vi "TB-Config.vi"(0 "Params":T27={"Low cutoff (kHz)"=0.0, "High cutoff (kHz)"=0.0, "Duration (min)"=0.0, "dB SPL"=0.0, "Waveform"=enum."OFF", "WAVfile"=path "", "refWav"=path "", "use mic correction"=FALSE, "micCorrFile"=path "", "Pistonphone Level (dB SPL)"=0.0, "Sampling rate (Hz)"=0.0, "Buffer length (s)"=0.0, "Stream mic"=FALSE, "Fine adjust"={"Max"=0.0, "Min"=0.0}, "Mic gain"=0.0, "atten"=0.0, "resol (Hz)"=0.0, "navgs"=0, "Allow Slack"=FALSE, "max starts"=0, "Freq (kHz)"=8.0, "Tma (s)"=0.0, "Streamed"=[], "Drive"=""}, 1 "Exposure?":bool, 9 "ID":string, 11 "error in (no error)":errorcluster) -> (4 "state":T25, 10 "Num Buffers":i32, 13 "stimulus state":T1, 14 "StimChan":T24 {"Filter"."IIR Filter Cluster"."Forward Coefficients" format="%.4f"; "Filter"."IIR Filter Cluster"."Reverse Coefficients" format="%.4f"}, 15 "error out":errorcluster)   [LabVIEW 2020]
uses:
  Typedefs/TB-Parameters.ctl
  epl-vi-lib/Signal Synthesis VIs/Controls/Waveform XCtl/Waveform Enum.ctl
  Typedefs/TB-Runtime state.ctl
  <vilib>/sound2/lvsound2.llb/Sound File Refnum.ctl
  Typedefs/TB-Setup Log.ctl
  epl-vi-lib/Signal Synthesis VIs/Controls/Waveform XCtl/Waveform Data.ctl
  epl-vi-lib/Signal Synthesis VIs/Waveform VIs/Tone VIs/Tone Params.ctl
  epl-vi-lib/Signal Synthesis VIs/Waveform VIs/Pulse Train VIs/Pulse Train Params.ctl
  epl-vi-lib/Signal Synthesis VIs/Waveform VIs/Pulse Train VIs/Pulse Polarity.ctl
  epl-vi-lib/Signal Synthesis VIs/Waveform VIs/Pulse Train VIs/PT-Continuous State.ctl
  epl-vi-lib/Signal Synthesis VIs/Waveform VIs/Noise VIs/Noise Params.ctl
  epl-vi-lib/Signal Synthesis VIs/Waveform VIs/File VIs/StimFile-Params.ctl
  epl-vi-lib/Signal Synthesis VIs/Waveform VIs/FM Sweep VIs/FM Sweep Params.ctl
  epl-vi-lib/Signal Synthesis VIs/Waveform VIs/Chirp Train VIs/Chirp Train.ctl
  epl-vi-lib/Signal Synthesis VIs/Waveform VIs/Chirp Train VIs/Chirp Train Params.ctl
  epl-vi-lib/Signal Synthesis VIs/Waveform VIs/Complex Tone VIs/CT-Params.ctl
  epl-vi-lib/Signal Synthesis VIs/Waveform VIs/Complex Tone VIs/CT-Phase Enum.ctl
  epl-vi-lib/Signal Synthesis VIs/Waveform VIs/Complex Tone VIs/CT-Runtime Data.ctl
  epl-vi-lib/Signal Synthesis VIs/Waveform VIs/Moving Ripple VIs/Moving Ripple.ctl
  epl-vi-lib/Signal Synthesis VIs/Waveform VIs/Moving Ripple VIs/Moving Ripple.Params.ctl
  epl-vi-lib/Signal Synthesis VIs/Waveform VIs/Moving Ripple VIs/Moving Ripple.Data.ctl
  epl-vi-lib/Signal Synthesis VIs/Controls/Filter XCtl/Filter Data.ctl
  epl-vi-lib/Signal Synthesis VIs/Controls/Gate XCtl/Gate Data.ctl
  epl-vi-lib/Signal Synthesis VIs/Controls/Level XCtl/Level Data.ctl
  epl-vi-lib/Signal Synthesis VIs/Controls/Level XCtl/Level Units.ctl
  Typedefs/TB-Stimulus State.ctl
  epl-vi-lib/Connection VIs/Type Defs/Input sources.ctl
  epl-vi-lib/Connection VIs/Type Defs/Output sources.ctl
  epl-vi-lib/Utility VIs/Math VIs/dB to Linear (scalar).vi
  epl-vi-lib/Utility VIs/Array Manipulation VIs/Sort and Index (I32).vi
  epl-vi-lib/Signal Synthesis VIs/Controls/Waveform XCtl/Waveform XCtl.xctl
  epl-vi-lib/Signal Synthesis VIs/Controls/Filter XCtl/Filter XCtl.xctl
  epl-vi-lib/Signal Synthesis VIs/Controls/Gate XCtl/Gate Control.xctl
  epl-vi-lib/Signal Synthesis VIs/Controls/Level XCtl/Level XCtl.xctl
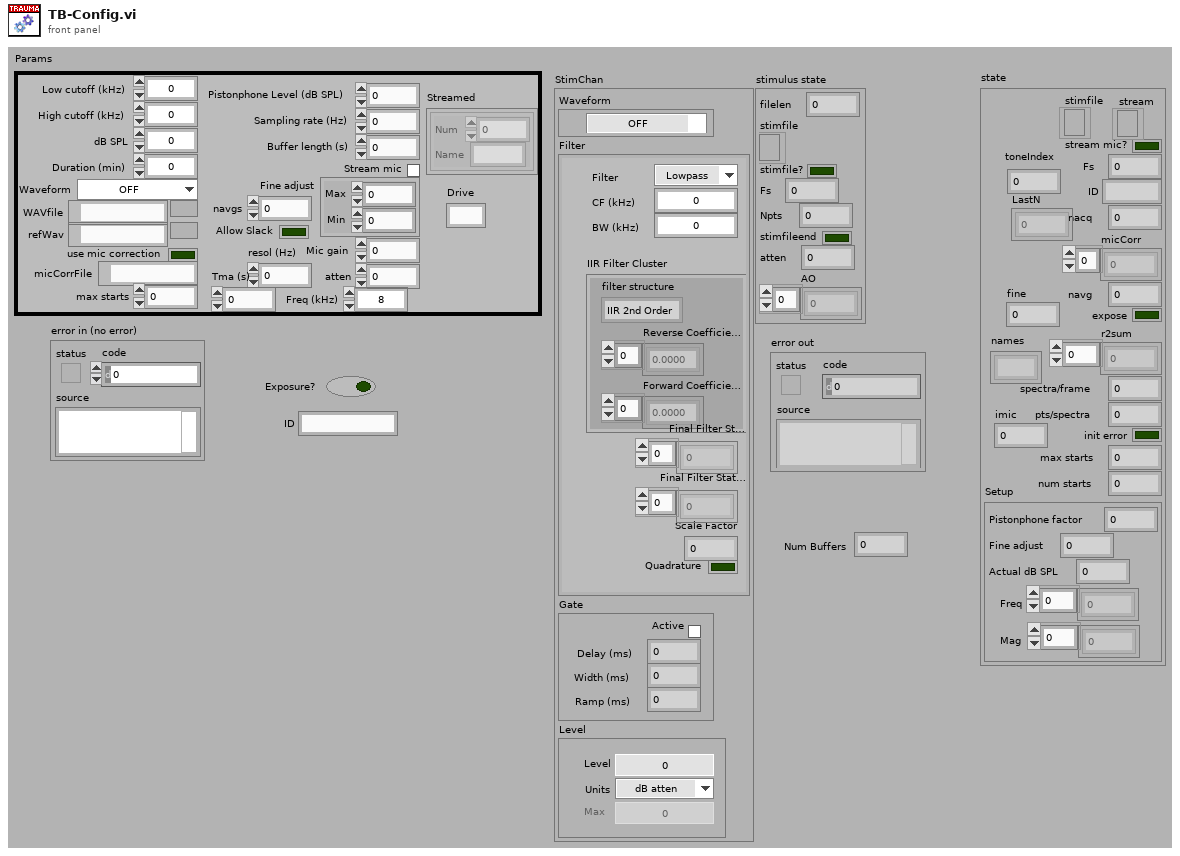
[diagram p1: front panel]
types:
  T1 = typedef "TB-Stimulus State.ctl" = cluster{"filelen":i32, "stimfile":T2, "stimfile?":bool, "Fs":dbl, "Npts":i32, "stimfileend":bool, "atten":dbl, "AO":i32[]}
  T2 = typedef "Sound File Refnum.ctl" = refnum<file>
  T3 = typedef "Waveform XCtl.xctl/Waveform Data.ctl" = cluster{"Type":T4, "Tone":T5, "Pulse Train":T6, "Noise":T9, "File":T10, "FMSweep":T11, "Chirp Train":T12, "Complex Tone":cluster{"Params":T14, "Data":T16}, "Moving Ripple":T17}
  T4 = typedef "Waveform Enum.ctl" = enum16{"OFF", "Tone", "Noise", "Pulse Train", "File", "FM Sweep", "Chirp Train", "Complex Tone", "FM Tone", "Moving Ripple"}
  T5 = typedef "Tone Params.ctl" = cluster{"Frequency (kHz)":dbl, "Last Freq":dbl, "Last Phase":dbl}
  T6 = typedef "Pulse Train Params.ctl" = cluster{"Pulse width (us)":dbl, "Pulse rate (Hz)":dbl, "Gap (ms)":dbl, "Polarity":T7, "PT State":T8, "Asynch":bool}
  T7 = typedef "Pulse Polarity.ctl" = enum16{"POS", "NEG", "POS-NEG", "NEG-POS"}
  T8 = typedef "PT-Continuous State.ctl" = cluster{"Template":dbl[], "Nperiod":i32, "Index":i32, "Pulse Rate (Hz)":dbl, "Phase (cycles)":dbl, "Noff":i32}
  T9 = typedef "Noise Params.ctl" = cluster{"InvFilt":bool, "Noise":dbl[], "CurPt":i32, "Aweight":bool, "Seed":i32, "afile":path}
  T10 = typedef "StimFile-Params.ctl" = cluster{"Filename":path, "Signal":dbl[], "Channel":i32, "stream":bool, "offset":i32, "nreps":i32, "loops":i32, "Randomize":bool, "order":i32[], "Seed":i32, "Tokens":i32}
  T11 = typedef "FM Sweep Params.ctl" = cluster{"Rate (oct/s)":dbl, "Fmin (Hz)":dbl, "Fmax (Hz)":dbl, "Ramp (ms)":dbl, "Linear":bool}
  T12 = typedef "Chirp Train.ctl" = cluster{"Params":T13, "Data":cluster{"WF":dbl[]}}
  T13 = typedef "Chirp Train Params.ctl" = cluster{"Fmin (kHz)":dbl, "Fmax (kHz)":dbl, "Compensate":bool, "Duration (ms)":dbl}
  T14 = typedef "CT-Params.ctl" = cluster{"F0 (Hz)":dbl, "Band":cluster{"Flow (Hz)":dbl, "Fhigh (Hz)":dbl}, "Phase":T15, "Min F0 (Hz)":dbl, "Max F0 (Hz)":dbl, "ContinRandPhase":bool, "Max peak factor":dbl, "Max mod depth":dbl, "MinHarmNum":i32, "MaxHarmNum":i32, "Level Mode":enum16{"per component", "overall rms"}, "% jitter":dbl}
  T15 = typedef "CT-Phase Enum.ctl" = enum16{"Cosine", "Random", "Alternating"}
  T16 = typedef "CT-Runtime Data.ctl" = cluster{"Ncomp":i32, "MinHarm":i32, "Phase":dbl[], "Amplitude":dbl[], "Npts/frame":i32, "Last F0":dbl, "Fmin":dbl, "Fmax":dbl, "Lslope":dbl, "randphase":bool, "overall rms":bool, "fmult":dbl[], "jittered":bool}
  T17 = typedef "Moving Ripple.ctl" = cluster{"Params":T18, "Data":T19}
  T18 = typedef "Moving Ripple.Params.ctl" = cluster{"Fmin":dbl, "Fmax":dbl, "Density":dbl, "Velocity":dbl, "Depth":dbl, "Phase":dbl, "Comp/oct":i32}
  T19 = typedef "Moving Ripple.Data.ctl" = cluster{"Freq":dbl[], "A":dbl[], "phase":dbl[], "Phase":dbl}
  T20 = typedef "Filter XCtl.xctl/Filter Data.ctl" = cluster{"CF (kHz)":dbl, "BW (kHz)":dbl, "IIR Filter Cluster":cluster{"filter structure":enum32{"IIR 2nd Order", "IIR 4th Order"}, "Reverse Coefficients":dbl[], "Forward Coefficients":dbl[]}, "Final Filter State":dbl[], "Scale Factor":dbl, "Final Filter State 2":dbl[], "Quadrature":bool, "Type":enum16{"Lowpass", "Highpass", "Bandpass", "Bandstop", "OFF"}}
  T21 = typedef "Gate Control.xctl/Gate Data.ctl" = cluster{"Active":bool, "Delay (ms)":dbl, "Width (ms)":dbl, "Ramp (ms)":dbl}
  T22 = typedef "Level XCtl.xctl/Level Data.ctl" = cluster{"Level":dbl, "Units":T23, "Max":dbl, "Multiplier":dbl, "Cal File":path, "Cal":cluster{"Freq (Hz)":dbl[], "Mag (dB SPL)":dbl[], "Phase (deg)":dbl[]}}
  T23 = typedef "Level Units.ctl" = enum16{"dB atten", "dB SPL", "dB re 1 Vrms", "dB V/Hz½", "mW", "dB HL", "Volts", "dB mW"}
  T24 = cluster{"Waveform":T3, "Filter":T20, "Gate":T21, "Level":T22}
  T25 = typedef "TB-Runtime state.ctl" = cluster{"stimfile":T2, "stream mic?":bool, "Fs":dbl, "ID":string, "micCorr":dbl[], "navg":i32, "r2sum":dbl[], "expose":bool, "spectra/frame":i32, "pts/spectra":i32, "nacq":i32, "init error":bool, "max starts":i32, "num starts":i32, "Setup":T26, "toneIndex":i32, "LastN":dbl[], "fine":dbl, "imic":i32, "stream":refnum<file>, "names":string[]}
  T26 = typedef "TB-Setup Log.ctl" = cluster{"Pistonphone factor":dbl, "Fine adjust":dbl, "Actual dB SPL":dbl, "Freq":dbl[], "Mag":dbl[]}
  T27 = typedef "TB-Parameters.ctl" = cluster{"Low cutoff (kHz)":dbl, "High cutoff (kHz)":dbl, "Duration (min)":dbl, "dB SPL":dbl, "Waveform":T4, "WAVfile":path, "refWav":path, "use mic correction":bool, "micCorrFile":path, "Pistonphone Level (dB SPL)":dbl, "Sampling rate (Hz)":dbl, "Buffer length (s)":dbl, "Stream mic":bool, "Fine adjust":cluster{"Max":dbl, "Min":dbl}, "Mic gain":dbl, "atten":dbl, "resol (Hz)":dbl, "navgs":i32, "Allow Slack":bool, "max starts":i32, "Freq (kHz)":dbl, "Tma (s)":dbl, "Streamed":cluster{"Num":i32, "Name":string}[], "Drive":string}
  T28 = typedef "Output sources.ctl" = u16
  T29 = typedef "Input sources.ctl" = u16
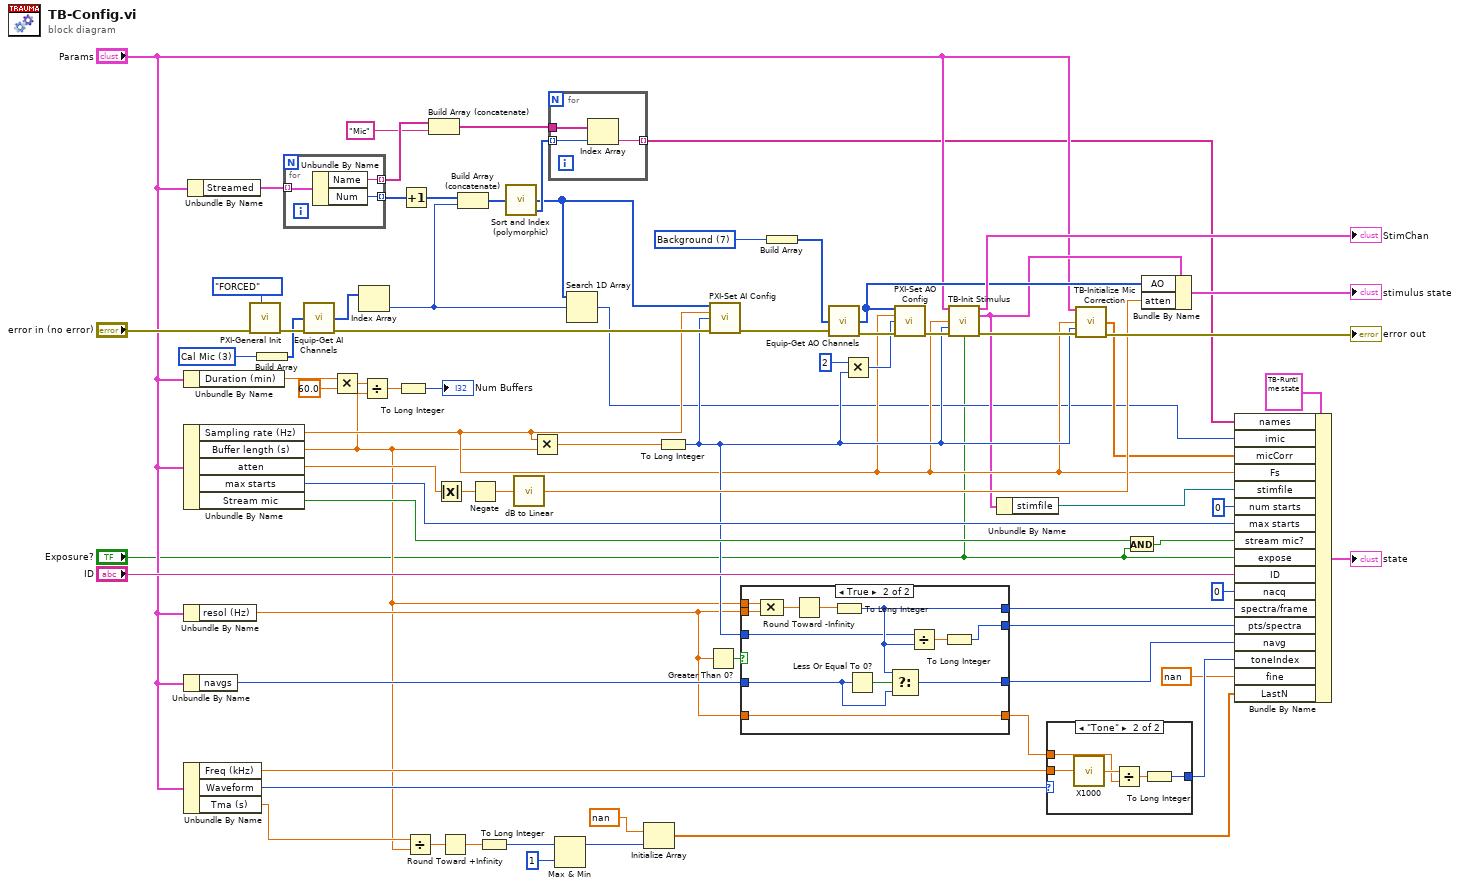
[diagram p0: block diagram]
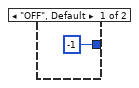
[diagram p2: hidden frame]
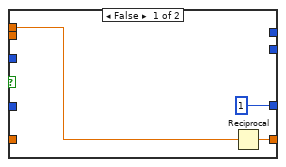
[diagram p3: hidden frame]
diagram:
  w56 = T28 7 items=["--unused--", "Right primary", "Right secondary", "Left primary", "Left secondary", "Shocks", "Startle", "Background", "Shaker"] ("Ring")
  w57 = T29 3 items=["--unused--", "Probe Mic Right", "Probe Mic Left", "Cal Mic", "ABR", "CAP Right", "CAP Left", "Startle piezo", "Temperature", "Heart rate", "Accelerometer"] ("Ring")
  n1 = Unbundle By Name("Params") -> ("Duration (min)"=w63:dbl)
  n2 = Unbundle By Name("Params") -> ("Sampling rate (Hz)"=w35:dbl, "Buffer length (s)"=w25:dbl, "atten"=w44:dbl, "max starts"=w42:i32, "Stream mic"=w43:bool)
  n3 = Unbundle By Name("Params") -> ("resol (Hz)"=w29:dbl)
  n4 = Unbundle By Name("Params") -> ("navgs"=w46:i32)
  n5 = Unbundle By Name("Params") -> ("Freq (kHz)"=w27:dbl, "Waveform"=w31:T4, "Tma (s)"=w26:dbl)
  n6 = Unbundle By Name("Params") -> ("Streamed"=w15:cluster{"Num":i32, "Name":string}[])
  n7 = call "PXI-General Init.vi"("Double Buffer Mode"=enum32{"OFF", "ENABLED", "FORCED"}."FORCED", "error in (no error)"="error in (no error)") -> ("error out"=w73:errorcluster)  [unwired: 9 in]
  n8 = Build Array(w57) -> (w72:T29[])
  n9 = for {
    tunnel: w15 -> [w79] mode=indexing
    tunnel: [w78] -> w14 mode=indexing
    tunnel: [w77] -> w10 mode=indexing
    n10 = Unbundle By Name(w79) -> ("Name"=w77:string, "Num"=w78:i32)
  }
  n11 = call "Equip-Get AI Channels.vi"("Inputs"=w72, "error in (no error)"=w73) -> ("AI Channels"=w13:i32[], "error out"=w68:errorcluster)  [unwired: 12 in]
  n12 = Multiply(x=w63, y=60.0) -> (x*y=w61:dbl)
  n13 = Index Array(array=w13) -> (element=w5:i32)  [unwired: 1 in]
  n14 = Divide(x=w61, y=w25) -> (x/y=w60:dbl)
  n15 = To Long Integer(number=w60) -> (32bit integer=→"Num Buffers":i32)
  n16 = Increment(x=w14) -> (x+1=w12:i32[])
  n17 = Divide(x=w26, y=w25) -> (x/y=w24:dbl)
  n18 = Build Array (concatenate)(w10, "Mic") -> (w8:string[])
  n19 = Absolute Value(x=w44) -> (abs(x)=w51:dbl)
  n20 = Round Toward +Infinity(x=w24) -> (ceil(x): smallest int >= x=w23:dbl)
  n21 = Build Array (concatenate)(w12, w5) -> (w11:i32[])
  n22 = Negate(x=w51) -> (-x=w50:dbl)
  n23 = To Long Integer(number=w23) -> (32bit integer=w22:i32)
  n24 = call-poly "Sort and Index (polymorphic).vi"("X"=w11) -> ("Index"=w7:i32[], "Sort(X)"=w6:i32[])  [unwired: 3 in]
  n25 = call-poly "dB to Linear.vi"("dB"=w50) -> ("linear"=w40:dbl)
  n26 = Multiply(x=w35, y=w25) -> (x*y=w70:dbl)
  n27 = for {
    tunnel: w8 -> [w82]
    tunnel: w7 -> [w81] mode=indexing
    tunnel: [w80] -> w3 mode=indexing
    n28 = Index Array(array=w82, index=w81) -> (element=w80:string)
  }
  n29 = Max & Min(x=w22, y=1) -> (max(x,y)=w18:i32)  [unwired: 1 out]
  n30 = Search 1D Array(1D array=w6, element=w5) -> (index of element=w4:i32)  [unwired: 1 in]
  n31 = Initialize Array(nan, w18) -> (w20:dbl[])
  n32 = To Long Integer(number=w70) -> (32bit integer=w37:i32)
  n33 = Greater Than 0?(x=w29) -> (x > 0?=w47:bool)
  n34 = call "PXI-Set AI Config.vi"("AI Channels"=w6, "Sampling Rate (Hz)"=w35, "Buffer Size"=w37, "error in (no error)"=w68) -> ("error out"=w65:errorcluster)  [unwired: 11 in]
  n35 = case shown="True" w47 {
    tunnel: w29 -> [_ w97]
    tunnel: w37 -> [_ w87]
    tunnel: w25 -> [w84 w94]
    tunnel: [_ w89] -> w49
    tunnel: [_ w92] -> w48
    tunnel: w46 -> [_ w90]
    tunnel: [1 ("navgs") w88] -> w45
    tunnel: [w83 w86] -> w28
    tunnel: w29 -> [_ w86]
    frame False {
      n36 = Reciprocal(x=w84) -> (1/x=w83:dbl)
    }
    frame True {
      n37 = Compound Arithmetic op=MULTIPLY(w94, w97) -> (w96:dbl)
      n38 = Round Toward -Infinity(1:w96) -> (0:w95:dbl)
      n39 = To Long Integer(number=w95) -> (32bit integer=w89:i32)
      n40 = Less Or Equal To 0?(x=w90) -> (x <= 0?=w91:bool)
      n41 = Select(t=w89, s=w91, f=w90) -> (s? t:f=w88:i32)
      n42 = Divide(x=w87, y=w89) -> (x/y=w93:dbl)
      n43 = To Long Integer(number=w93) -> (32bit integer=w92:i32)
    }
  }
  n44 = Build Array(w56) -> (w71:T28[])
  n45 = call "Equip-Get AO Channels.vi"("Outputs"=w71, "error in (no error)"=w65) -> ("AO Channels"=w39:i32[], "error out"=w67:errorcluster)  [unwired: 12 in]
  n46 = Multiply(x=2, y=w37) -> (x*y=w66:i32)
  n47 = call "PXI-Set AO Config.vi"("AO Channels"=w39, "Sampling Rate (Hz)"=w35, "Buffer Size"=w66, "error in (no error)"=w67) -> ("error out"=w64:errorcluster)  [unwired: 11 in]
  n48 = call "TB-Init Stimulus.vi"("Exposure parameters"="Params", "Sampling rate (Hz)"=w35, "Npts"=w37, "error in (no error)"=w64, "Exposure"="Exposure?") -> ("StimChan"=→"StimChan":T24, "stimulus state"=w34:T1, "error out"=w75:errorcluster)  [unwired: 8 in]
  n49 = Unbundle By Name(w34) -> ("stimfile"=w32:T2)
  n50 = case shown="\"Tone\"" w31 {
    tunnel: [-1 w99] -> w30
    tunnel: w28 -> [_ w101]
    tunnel: w27 -> [_ w103]
    frame "OFF", Default {
    }
    frame "Tone" {
      n51 = call "X1000.vi"("X"=w103) -> ("X/1000"=w102:dbl)
      n52 = Divide(x=w102, y=w101) -> (x/y=w100:dbl)
      n53 = To Long Integer(number=w100) -> (32bit integer=w99:i32)
    }
  }
  n54 = call "TB-Initialize Mic Correction.vi"("Exposure parameters"="Params", "Sampling rate (Hz)"=w35, "Npts"=w37, "error in (no error)"=w75) -> ("micCorr"=w36:dbl[], "error out"=→"error out":errorcluster)  [unwired: 10 in]
  n55 = And(x=w43, y="Exposure?") -> (x .and. y?=w2:bool)
  n56 = Bundle By Name(cluster=w34, "AO"=w39, "atten"=w40) -> (→"stimulus state":T1)
  n57 = Bundle By Name(cluster=T25 {"stimfile"=refnum, "stream mic?"=FALSE, "Fs"=0.0, "ID"="", "micCorr"=[], "navg"=0, "r2sum"=[], "expose"=FALSE, "spectra/frame"=0, "pts/spectra"=0, "nacq"=0, "init error"=FALSE, "max starts"=0, "num starts"=0, "Setup"={"Pistonphone factor"=0.0, "Fine adjust"=0.0, "Actual dB SPL"=0.0, "Freq"=[], "Mag"=[]}, "toneIndex"=0, "LastN"=[], "fine"=0.0, "imic"=0, "stream"=refnum, "names"=[]} ("state"), "names"=w3, "imic"=w4, "micCorr"=w36, "Fs"=w35, "stimfile"=w32, "num starts"=0, "max starts"=w42, "stream mic?"=w2, "expose"="Exposure?", "ID"="ID", "nacq"=0 ("navg"), "spectra/frame"=w49, "pts/spectra"=w48, "navg"=w45, "toneIndex"=w30, "fine"=nan, "LastN"=w20) -> (→"state":T25)
